vi "INI_Rebuild Property Files.vi"() -> (3 "Rebuild Property Files":bool)   [LabVIEW 2023]
doc: "Check to see if LV ini settings indicate scripting or private methods have been turned on since the BundleMagic help files were built."
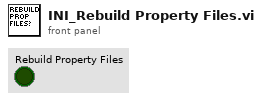
[diagram p1: front panel]
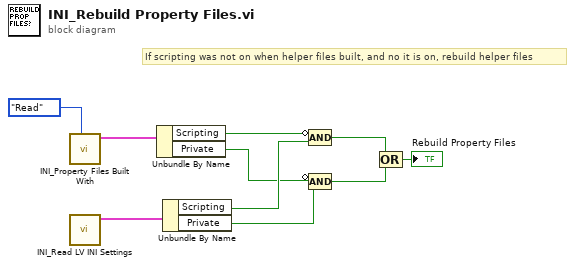
[diagram p0: block diagram]
diagram:
  # "If scripting was not on when helper files built, and no it is on, rebuild helper files"
  n1 = call "INI_Property Files Built With.vi"("File Action"=enum16{"Read", "Write"}."Read") -> ("Property Files Built With"=w9:cluster{"Scripting":bool, "Private":bool})  [unwired: 10 in]
  n2 = call "INI_Read LV INI Settings.vi"() -> ("LabVIEW INI Settings"=w8:cluster{"Scripting":bool, "Private":bool})  [unwired: 10 in, 1 out]
  n3 = Unbundle By Name(w9) -> ("Scripting"=w7:bool, "Private"=w5:bool)
  n4 = Unbundle By Name(w8) -> ("Scripting"=w6:bool, "Private"=w4:bool)
  n5 = Compound Arithmetic op=AND(invert w7, w6) -> (w3:bool)
  n6 = Compound Arithmetic op=AND(invert w5, w4) -> (w2:bool)
  n7 = Compound Arithmetic op=OR(w3, w2) -> (→"Rebuild Property Files":bool)
